vi "Test PINGREQ packet.vi"(8 "error in (no error)":errorcluster) -> (0 "error out":errorcluster)   [LabVIEW 2013]
uses:
  source/Control Packets/PINGREQ/PINGREQ.lvclass
  source/Control Packets/ControlPacket/ControlPacket.lvclass/ControlPacket.ctl
  source/Control Packets/ControlPacket/ControlPacket.lvclass
  <vilib>/addons/_JKI Toolkits/Caraya/classes/Test/Test.lvclass
  <vilib>/addons/_JKI Toolkits/Caraya/classes/Assert/Assert.lvclass
panel:
  out "Packet ID":u16 format="%04x"
  out "Absence of Packet Identifier":bool
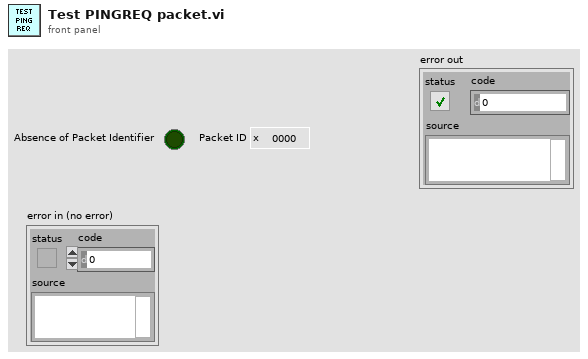
[diagram p1: front panel]
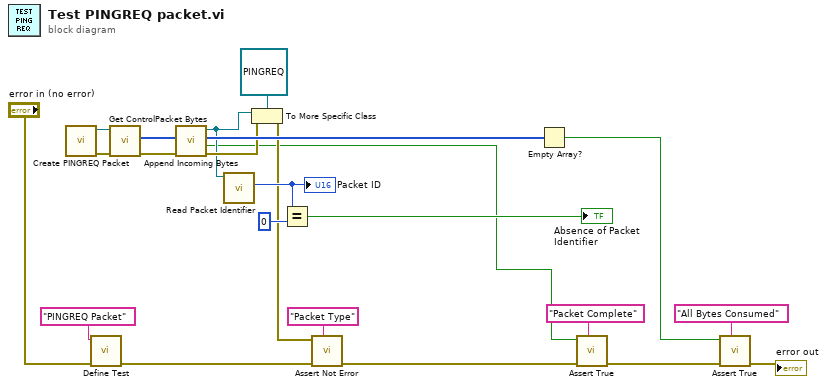
[diagram p0: block diagram]
diagram:
  n1 = call "Create PINGREQ Packet.vi"() -> ("error out"=w14:errorcluster, "PINGREQ out"=w15:refnum<class "PINGREQ.lvclass">)  [unwired: 10 in]
  n2 = call <vilib>:"Define Test.vi"("error in (no error)"="error in (no error)", "Label (VI Title)"="PINGREQ Packet") -> ("error out"=w9:errorcluster)  [unwired: 9 in]
  n3 = call "Get ControlPacket Bytes.vi"("error in (no error)"=w14, "ControlPacket"=w15) -> ("error out"=w21:errorcluster, "Bytes Stream"=w23:u8[])  [unwired: 6 in, 2 out]
  n4 = call "Append Incoming Bytes.vi"("error in (no error)"=w21, "Incoming Packets"=w23) -> ("error out"=w20:errorcluster, "Complete Packet"=w3:bool, "Remaining Packets"=w22:u8[], "ControlPacket"=w17:refnum<class "ControlPacket.lvclass">)  [unwired: 6 in]
  n5 = call "Read Packet Identifier.vi"("ControlPacket in"=w17) -> ("Packet Identifier"=w19:u16)  [unwired: 9 in, 1 out]
  "Packet ID" <- w19
  n6 = To More Specific Class(target class=refnum<class "PINGREQ.lvclass"> refnum ("MQTT_Control_Packets.lvlib:PINGREQ.lvclass"), reference=w17, error in=w20) -> (error out=w6:errorcluster)  [unwired: 1 out]
  n7 = Equal?(x=w19, y=u16 0) -> (x = y?=→"Absence of Packet Identifier":bool)
  n8 = call <vilib>:"Assert Not Error.vi"("Label"="Packet Type" ("Label (VI Title)"), "error in (no error)"=w9, "Not Error?"=w6) -> ("error out"=w1:errorcluster)  [unwired: 8 in]
  n9 = Empty Array?(array=w22) -> (empty?=w2:bool)
  n10 = call <vilib>:"Assert True.vi"("Label"="Packet Complete" ("Label (VI Title)"), "error in (no error)"=w1, "True?"=w3) -> ("error out"=w7:errorcluster)  [unwired: 8 in]
  n11 = call <vilib>:"Assert True.vi"("Label"="All Bytes Consumed" ("Label (VI Title)"), "error in (no error)"=w7, "True?"=w2) -> ("error out"=→"error out":errorcluster)  [unwired: 8 in]
